vi "Cook Next Recipe Step.vi"(8 "error in (no error)":errorcluster, 11 "Cooker Actor in":refnum<class "Cooker Actor.lvclass">) -> (0 "error out":errorcluster, 3 "Cooker Actor out":refnum<class "Cooker Actor.lvclass">)   [LabVIEW 2024, in "Cooker Actor.lvlib" / "Cooker Actor.lvclass"]
uses:
  Cooker Actor.lvclass
  Cooker Actor.lvclass/Cooker Actor.ctl
  <vilib>/ActorFramework/Message Enqueuer/Message Enqueuer.lvclass/Message Enqueuer.ctl
  Oven Actor/Oven Actor Messages/Apply Heat Msg/Apply Heat Msg.lvclass/Apply Heat Msg.ctl
  Timer Actor/Timer Actor Messages/Start Count Down Msg/Start Count Down Msg.lvclass/Start Count Down Msg.ctl
  <vilib>/ActorFramework/Message Enqueuer/Enqueue.vi
  Recipe Actor/Recipe Actor Messages/Get Next Step Msg/Get Next Step Msg.lvclass
  C:/Program Files/National Instruments/LabVIEW 2024/vi.lib/ActorFramework/Message/Message.lvclass
  Oven Actor/Oven Actor Messages/Apply Heat Msg/Apply Heat Msg.lvclass
  Timer Actor/Timer Actor Messages/Start Count Down Msg/Start Count Down Msg.lvclass
  <vilib>/ActorFramework/Message Priority Queue/Priority Enqueue.vi
  Recipe Actor/Recipe Step/Recipe Step.lvclass
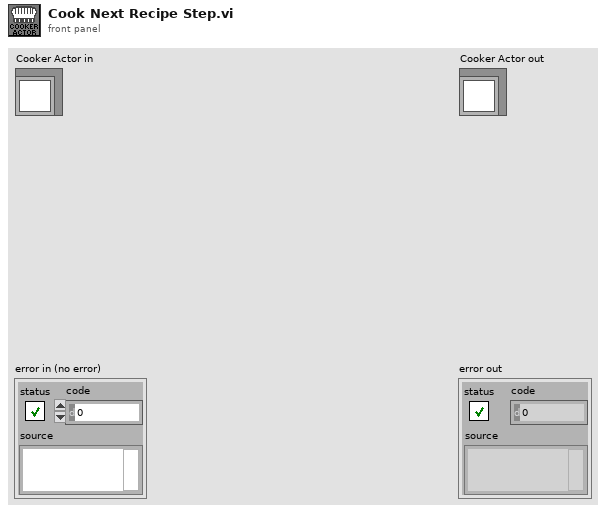
[diagram p1: front panel]
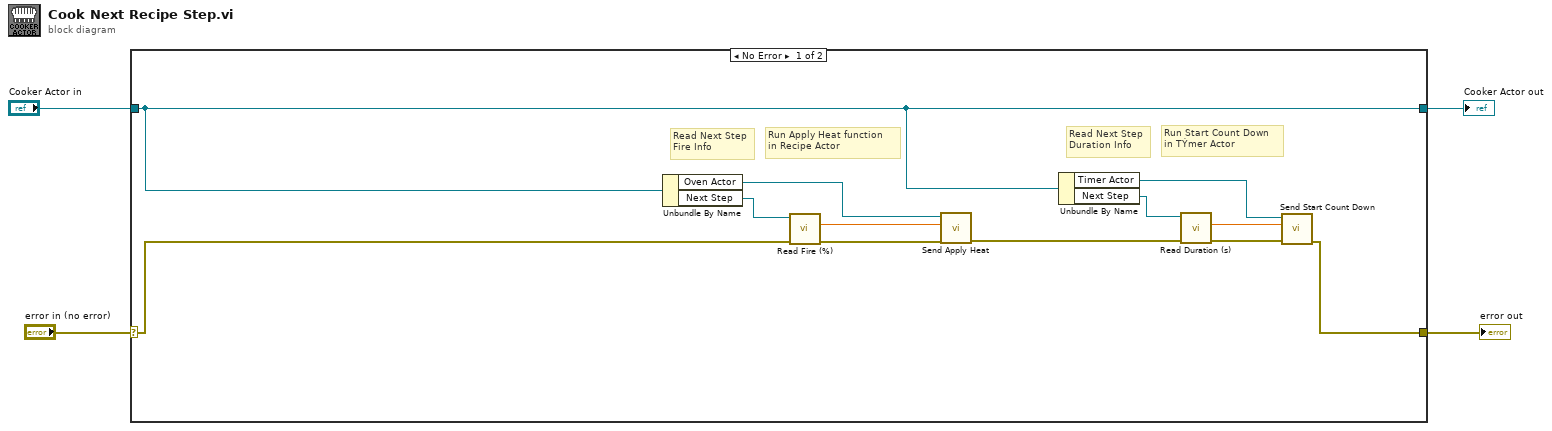
[diagram p0: block diagram]
diagram:
  n1 = case shown="No Error" "error in (no error)" {
    selector: "error in (no error)" -> [w16 w18]
    tunnel: [w6 w18] -> w3
    tunnel: [w5 w17] -> w1
    tunnel: "Cooker Actor in" -> [w5 w17]
    frame No Error {
      # "Run Start Count Down\nin TÝmer Actor"
      # "Read Next Step\nDuration Info"
      # "Run Apply Heat function\nin Recipe Actor"
      # "Read Next Step\nFire Info"
      n2 = Unbundle By Name(w5) -> ("Oven Actor"=w12:refnum<class "Message Enqueuer.lvclass">, "Next Step"=w15:refnum<class "Recipe Step.lvclass">)
      n3 = call-dynamic "Read Fire (%).vi"("error in (no error)"=w16, "Recipe Step in"=w15) -> ("error out"=w13:errorcluster, "Fire (%)"=w14:dbl)  [unwired: 7 in, 1 out]
      n4 = call "Send Apply Heat.vi"("error in (no error)"=w13, "Fire (%)"=w14, "Message Enqueuer"=w12) -> ("error out"=w11:errorcluster)  [unwired: 7 in, 1 out]
      n5 = Unbundle By Name(w5) -> ("Timer Actor"=w7:refnum<class "Message Enqueuer.lvclass">, "Next Step"=w10:refnum<class "Recipe Step.lvclass">)
      n6 = call-dynamic "Read Duration (s).vi"("error in (no error)"=w11, "Recipe Step in"=w10) -> ("error out"=w9:errorcluster, "Duration (s)"=w8:dbl)  [unwired: 7 in, 1 out]
      n7 = call "Send Start Count Down.vi"("error in (no error)"=w9, "Seconds To Wait"=w8, "Message Enqueuer"=w7) -> ("error out"=w6:errorcluster)  [unwired: 7 in, 1 out]
    }
    frame Error {
    }
  }
  "error out" <- w3
  "Cooker Actor out" <- w1
